vi "numlock flush.vi"(8 "error in (no error)":errorcluster, 11 "logger":T1) -> (0 "error out":errorcluster, 3 "logger out":T1)   [LabVIEW 2019]
uses:
  numlock.ctl
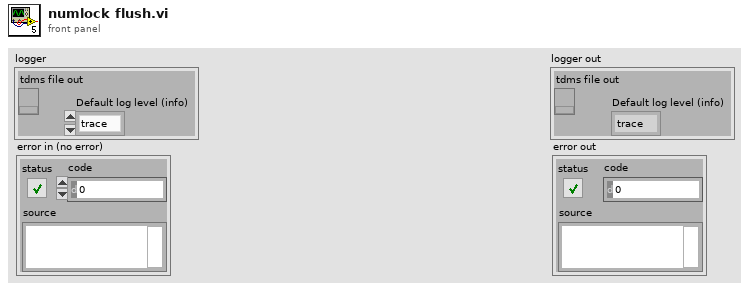
[diagram p1: front panel]
types:
  T1 = typedef "numlock.ctl" = cluster{"tdms file out":refnum<k34>, "Default log level (info)":enum16{"trace", "debug", "info", "warn", "error"}}
  T2 = enum16{"trace", "debug", "info", "warn", "error"}
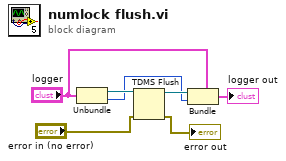
[diagram p0: block diagram]
diagram:
  n1 = Unbundle("logger") -> ("tdms file out"=w7:refnum<k34>, "Default log level (info)"=w4:T2)
  n2 = TDMS Flush(4:"error in (no error)", 7:w7) -> (0:→"error out":errorcluster, 3:w6:refnum<k34>)
  n3 = Bundle(cluster="logger", "tdms file out"=w6, "Default log level (info)"=w4) -> (→"logger out":T1)
